vi "yaokong 10.23.vi"(0 "串口设置（遥控器）":T1={"波特率"=115200, "数据位"=8, "校验"=enum."None", "停止位"=10, "流控制"=0} {"流控制" items=["无"=0, "XON/XOFF"=1, "RTS/CTS"=2, "DTR/DSR"=4]; "停止位" items=["1.0"=10, "1.5"=15, "2.0"=20]; "数据位" min=5 max=8 step=1; "波特率" items=["460800"=460800, "75"=75, "110"=110, "134"=134, "150"=150, "300"=300, "600"=600, "1200"=1200, "1800"=1800, "2400"=2400, "4800"=4800, "7200"=7200, "9600"=9600, "14400"=14400, "19200"=19200, "28800"=28800, "38400"=38400, "56000"=56000, "57600"=57600, "115200"=115200, "128000"=128000, "230400"=230400]}, 2 "串口选择":refnum<visa-resource-name>="ASRL5::INSTR" caption="VISA资源名称") -> (9 "遥控器数据模式":T2={"CH0"=1024, "CH1"=1024, "CH2"=1024, "CH3"=1024, "CH5"=1024, "CH4"=1024, "Key0"=FALSE, "Key1"=FALSE, "Key2"=FALSE, "Key3"=FALSE, "Key4"=FALSE} {"CH4" scale=0.0..2048.0; "CH5" scale=0.0..2048.0; "CH3" scale=0.0..2048.0; "CH2" scale=0.0..2048.0; "CH1" scale=0.0..2048.0; "CH0" scale=0.0..2048.0})   [LabVIEW 2016]
uses:
  <vilib>/Platform/TimedLoop/XDataNode/timing_clust.ctl
  <vilib>/Platform/TimedLoop/XDataNode/nitl_modes.ctl
  <vilib>/Platform/TimedLoop/XDataNode/wakeup.ctl
  <vilib>/Instr/_visa.llb/VISA Configure Serial Port (Instr).vi
  <vilib>/imath/engines/lvmath2/RunTimeEngine/BuiltInFunctions/length/NIMS_length(GV).vi
  <instcachedir>/0/NIMS_length(GV)_08A3D13377FD4E4B96F5795FBF3698FA.lvgen/NIMS_length(GV)_08A3D13377FD4E4B96F5795FBF3698FA_003.vi
  <vilib>/imath/engines/lvmath2/RunTimeEngine/RangeToken/NIMS_Range_R3 - Integer.vi
  <instcachedir>/0/NIMS_Range_R3 - Integer_A435E2FF893B4C718FD5055FE39FE2F6.lvgen/NIMS_Range_R3 - Integer_A435E2FF893B4C718FD5055FE39FE2F6_000.vi
  <vilib>/imath/engines/lvmath2/RunTimeEngine/CommandStatement/MC_CommandStatement_break.vi
  <vilib>/imath/engines/lvmath2/RunTimeEngine/IndexRead/NIMS V(S).vi
  <instcachedir>/0/NIMS V(S)_0488751826AF41519A22953C041130DC.lvgen/NIMS V(S)_0488751826AF41519A22953C041130DC_004.vi
  <vilib>/imath/engines/lvmath2/RunTimeEngine/ErrorHandling/NIMS_Create Error From Enums.vi
  <vilib>/imath/engines/lvmath2/RunTimeEngine/RowToken/NIMS_RowToken_M_SorRV.vi
  <instcachedir>/0/NIMS_RowToken_M_SorRV_4D710C5E6F8040F3A39B2F03436798DB.lvgen/NIMS_RowToken_M_SorRV_4D710C5E6F8040F3A39B2F03436798DB_001.vi
  <vilib>/imathl/engines/lvmath/Functions/Error Handling/Create Error.vi
  <vilib>/imath/engines/lvmath2/RunTimeEngine/BuiltInFunctions/length/NIMS_length(GM).vi
  <instcachedir>/0/NIMS_length(GM)_47CEC356FCE0482D9BA47DC61C99F2C7.lvgen/NIMS_length(GM)_47CEC356FCE0482D9BA47DC61C99F2C7_001.vi
  <vilib>/imath/engines/lvmath2/RunTimeEngine/IndexRead/NIMS M(S).vi
  <instcachedir>/0/NIMS M(S)_B826C018497E4940AE96BD27B540B6FB.lvgen/NIMS M(S)_B826C018497E4940AE96BD27B540B6FB_005.vi
  <vilib>/imath/engines/lvmath2/RunTimeEngine/BuiltInFunctions/is_empty/NIMS_is_empty(GV).vi
  <instcachedir>/0/NIMS_is_empty(GV)_FC7E7C3D9544432CB6AA2416ADCF6D56.lvgen/NIMS_is_empty(GV)_FC7E7C3D9544432CB6AA2416ADCF6D56_000.vi
  <vilib>/imath/engines/lvmath2/RunTimeEngine/BuiltInFunctions/int32/NIMS_int32(int).vi
  <instcachedir>/0/NIMS_int32(int)_E7E4C8D9008A4CBD9466BF2F069BABE1.lvgen/NIMS_int32(int)_E7E4C8D9008A4CBD9466BF2F069BABE1_000.vi
  <vilib>/imath/engines/lvmath2/RunTimeEngine/BuiltInFunctions/is_empty/NIMS_is_empty(GM).vi
  <instcachedir>/0/NIMS_is_empty(GM)_AF8F13F4B7FD436CB1855477E2504B8A.lvgen/NIMS_is_empty(GM)_AF8F13F4B7FD436CB1855477E2504B8A_004.vi
  <vilib>/imath/engines/lvmath2/RunTimeEngine/BuiltInFunctions/zeros/NIMS_M=zeros(I32,I32).vi
  <vilib>/imath/engines/lvmath2/RunTimeEngine/IndexRead/NIMS V(R2).vi
  <instcachedir>/0/NIMS V(R2)_C76619605A0E4E9F8B2FA9389712AC47.lvgen/NIMS V(R2)_C76619605A0E4E9F8B2FA9389712AC47_002.vi
  <vilib>/imath/engines/lvmath2/RunTimeEngine/IndexReplace/NIMS M(S,$)=V.vi
  <instcachedir>/0/NIMS M(S,$)=V_BCCFA522A894489B8FA760383D74A164.lvgen/NIMS M(S,$)=V_BCCFA522A894489B8FA760383D74A164_001.vi
  <vilib>/imath/engines/lvmath2/RunTimeEngine/IndexRead/NIMS M($,S).vi
  <instcachedir>/0/NIMS M($,S)_3E5749BBB62E49528D4765A77F1F6D98.lvgen/NIMS M($,S)_3E5749BBB62E49528D4765A77F1F6D98_002.vi
  <vilib>/imath/engines/lvmath2/RunTimeEngine/BuiltInFunctions/sets_unique/NIMS_sets_unique(GV).vi
  <instcachedir>/0/NIMS_sets_unique(GV)_E0D8B80906AB4C8F84772F5CCB3705F2.lvgen/NIMS_sets_unique(GV)_E0D8B80906AB4C8F84772F5CCB3705F2_006.vi
  <instcachedir>/0/NIMS_length(GV)_08A3D13377FD4E4B96F5795FBF3698FA.lvgen/NIMS_length(GV)_08A3D13377FD4E4B96F5795FBF3698FA_002.vi
  <vilib>/imath/engines/lvmath2/RunTimeEngine/BuiltInFunctions/zeros/NIMS_V=zeros(I32,I32).vi
  <vilib>/imath/engines/lvmath2/RunTimeEngine/RangeToken/NIMS_Range_R2 - Integer.vi
  <instcachedir>/0/NIMS_Range_R2 - Integer_89B873E74E6E489885E44F751DD9C6BF.lvgen/NIMS_Range_R2 - Integer_89B873E74E6E489885E44F751DD9C6BF_000.vi
  <instcachedir>/0/NIMS V(S)_0488751826AF41519A22953C041130DC.lvgen/NIMS V(S)_0488751826AF41519A22953C041130DC_002.vi
  <vilib>/imath/engines/lvmath2/RunTimeEngine/BuiltInFunctions/sum/NIMS_sum(GV).vi
  <instcachedir>/0/NIMS_sum(GV)_67F5EC36BC034E54A6BEC5B0673C00E5.lvgen/NIMS_sum(GV)_67F5EC36BC034E54A6BEC5B0673C00E5_000.vi
  <vilib>/imath/engines/lvmath2/RunTimeEngine/IndexReplace/NIMS V(S)=S.vi
  <instcachedir>/0/NIMS V(S)=S_57E16554CB8B4B90AAB163894F717546.lvgen/NIMS V(S)=S_57E16554CB8B4B90AAB163894F717546_000.vi
  <vilib>/imath/engines/lvmath2/RunTimeEngine/BuiltInFunctions/max/1 input/NIMS_max(RV).vi
  <instcachedir>/0/NIMS_max(RV)_237633DB1D604D5BA7001287DF3C7957.lvgen/NIMS_max(RV)_237633DB1D604D5BA7001287DF3C7957_000.vi
  <vilib>/imath/engines/lvmath2/RunTimeEngine/BuiltInFunctions/findnz/NIMS_[1o]_findnz(GRowV).vi
  <instcachedir>/0/NIMS_[1o]_findnz(GRowV)_1AF74843B4874134ADE908C0A4A72F3C.lvgen/NIMS_[1o]_findnz(GRowV)_1AF74843B4874134ADE908C0A4A72F3C_000.vi
  <vilib>/imath/engines/lvmath2/RunTimeEngine/IndexRead/NIMS M($,R2).vi
  <instcachedir>/0/NIMS M($,R2)_D9380E19261A4ADFB2D364AF6959C6EF.lvgen/NIMS M($,R2)_D9380E19261A4ADFB2D364AF6959C6EF_002.vi
  <vilib>/imath/engines/lvmath2/RunTimeEngine/BuiltInFunctions/median/NIMS_RRow=median(RM,I32).vi
  <vilib>/imath/engines/lvmath2/RunTimeEngine/BuiltInFunctions/int32/NIMS_int32(real).vi
  <instcachedir>/0/NIMS_int32(real)_9F6AE75EF4BE45429513317A1C5A7040.lvgen/NIMS_int32(real)_9F6AE75EF4BE45429513317A1C5A7040_002.vi
  <vilib>/imath/engines/lvmath2/RunTimeEngine/VariableToken/NIMS_VariableToken_CondDefined.vi
  <instcachedir>/0/NIMS_VariableToken_CondDefined_06E9DA95BD4D46A6BA55EC651A891960.lvgen/NIMS_VariableToken_CondDefined_06E9DA95BD4D46A6BA55EC651A891960_004.vi
  <vilib>/imath/engines/lvmath2/RunTimeEngine/NodeEndStatement/NIMS_NodeEndStatement_Get Vector.vi
  <instcachedir>/0/NIMS_NodeEndStatement_Get Vector_9E4547DF38A84F62A7E036B4CE3D251C.lvgen/NIMS_NodeEndStatement_Get Vector_9E4547DF38A84F62A7E036B4CE3D251C_002.vi
  <vilib>/imath/engines/lvmath/Functions/Error Handling/MergeErrorsWrapper.vi
  <vilib>/imath/engines/lvmath2/RunTimeEngine/NodeEndStatement/NIMS_NodeEndStatement_Output.vi
  <instcachedir>/0/NIMS_NodeEndStatement_Output_53EC0D466D134D7ABD903AC30B43404B.lvgen/NIMS_NodeEndStatement_Output_53EC0D466D134D7ABD903AC30B43404B_004.vi
  <instcachedir>/0/NIMS_NodeEndStatement_Output_53EC0D466D134D7ABD903AC30B43404B.lvgen/NIMS_NodeEndStatement_Output_53EC0D466D134D7ABD903AC30B43404B_010.vi
  <vilib>/imath/engines/lvmath2/RunTimeEngine/ErrorHandling/NIMS_Finalize Error.vi
  <vilib>/Platform/TimedLoop/XDataNode/XDataNode.xnode
  <vilib>/Platform/TimedLoop/XDataNode/XDNodeRunTimeDep.lvlib
panel:
  out "error out":errorcluster caption="错误输出"
  in  "遥控器数据队列名":string="Queue_RemoteCtler"
  out "CtlerFrameData":u8[](array[numeric])
  out "输出变量":i32
  in  "全局停止":bool
  out "Serial Settings:Number of Bytes at Serial Port":u32
  out "CtlerData":u8[](array[numeric])
  out "读取缓冲区":string
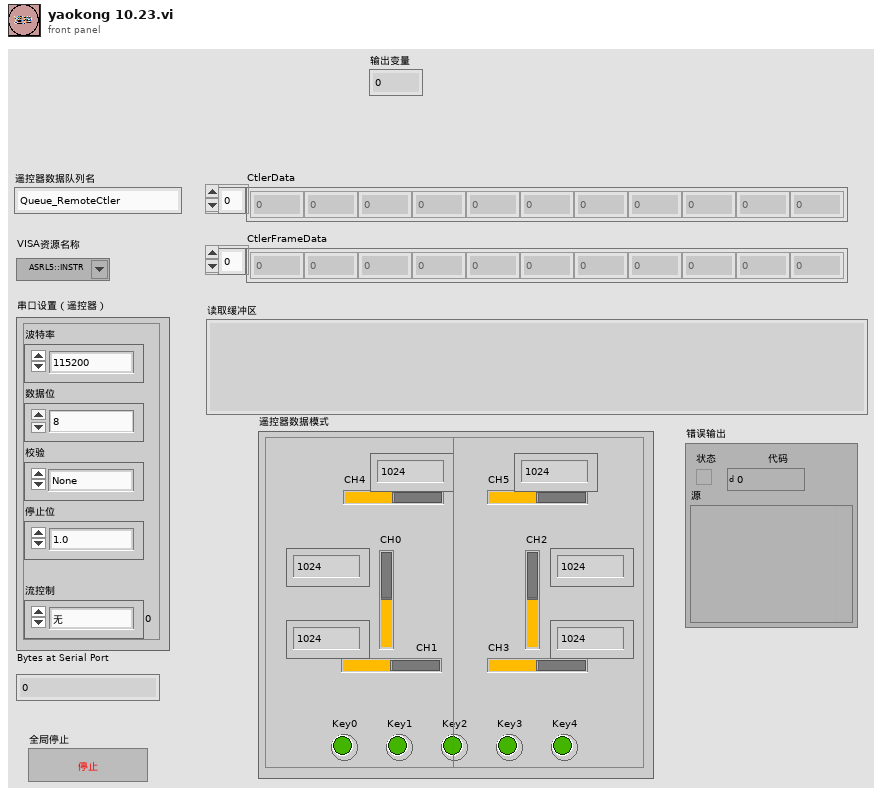
[diagram p1: front panel]
types:
  T1 = cluster{"波特率":u32, "数据位":u16, "校验":enum16{"None", "Odd", "Even", "Mark", "Space"}, "停止位":u16, "流控制":u16}
  T2 = cluster{"CH0":i32, "CH1":i32, "CH2":i32, "CH3":i32, "CH5":i32, "CH4":i32, "Key0":bool, "Key1":bool, "Key2":bool, "Key3":bool, "Key4":bool}
  T3 = typedef "XDNodeRunTimeDep.lvlib/timing_clust.ctl" = cluster{"Expected End [f-1]":u64, "Actual End [f-1]":u64, "Finished Late? [f-1]":bool, "Expected End [i-1]":u64, "Actual End [i-1]":u64, "Finished Late? [i-1]":bool, "Expected Start [i]":u64, "Actual Start [i]":u64, "Expected Start [f]":u64, "Actual Start [f]":u64, "Source Name":string, "Structure Name":string, "Period":i64, "Deadline":i64, "Offset":i64, "Start":i64, "Priority":i32, "Timeout":i32, "Mode":T4, "Wakeup Reason":T5, "Error":errorcluster, "Source Type":string, "Secondary Source Type":string, "Global End Time":u64, "Global Start Time":u64, "Frame Duration":u64, "Iteration Duration":u64, "Assigned CPU":i32, "I/O Scan Engine Mode":u32}
  T4 = typedef "XDNodeRunTimeDep.lvlib/nitl_modes.ctl" = enum32{"No Change", "Process missed periods, maintain original phase", "Discard missed periods, maintain original phase", "Process missed periods, ignore original phase", "Discard missed periods, ignore original phase"}
  T5 = typedef "XDNodeRunTimeDep.lvlib/wakeup.ctl" = enum32{"Normal", "Aborted", "Asynchronous wakeup", "Timing source error", "Timed loop error", "Timeout"}
  T6 = cluster{i32, i32, i32, i32, i32, i32, bool, bool, bool, bool, bool}
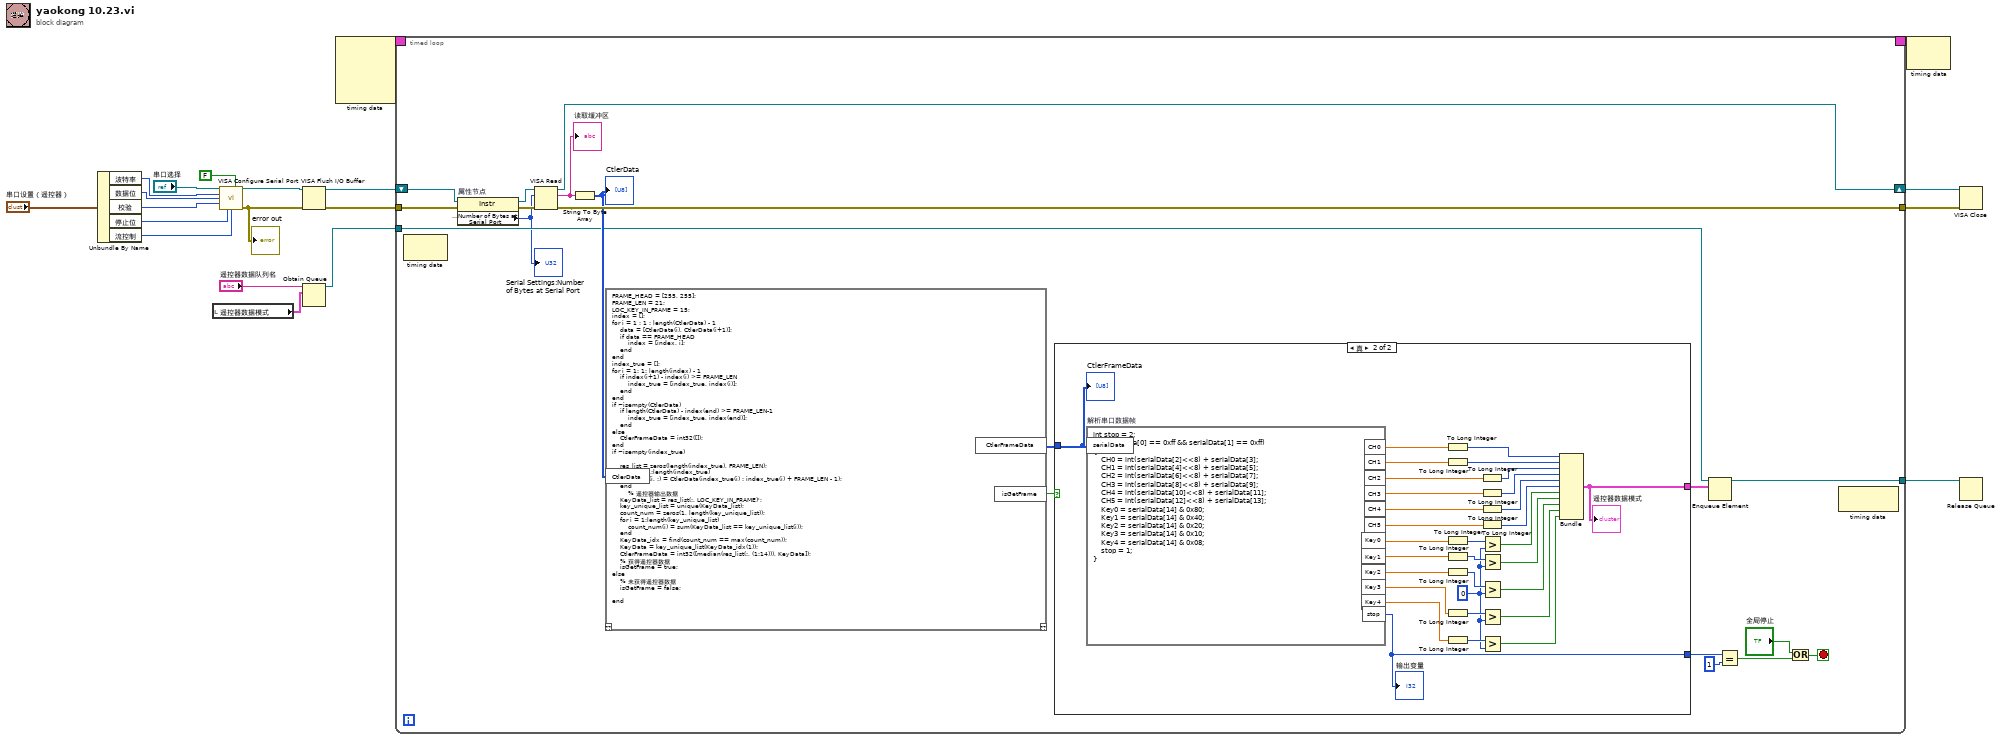
[diagram p0: block diagram]
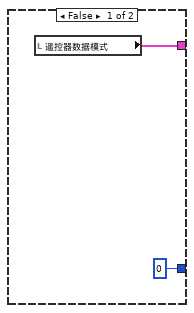
[diagram p2: hidden frame]
diagram:
  n1 = Unbundle By Name("串口设置（遥控器）") -> ("波特率"=w17:u32, "数据位"=w16:u16, "校验"=w15:enum16{"None", "Odd", "Even", "Mark", "Space"}, "停止位"=w14:u16, "流控制"=w13:u16)
  n2 = local read "遥控器数据模式"() -> (w6:T2)
  n3 = call-poly "VISA Configure Serial Port"("VISA resource name"="串口选择", "Enable Termination\nChar (T)"=FALSE ("Enable Termination\nChar (T)"), "baud rate (9600)"=w17, "data bits (8)"=w16, "parity (0:none)"=w15, "stop bits (10: 1 bit)"=w14, "flow control (0:none)"=w13) -> ("VISA resource name out"=w4:refnum<visa-resource-name>, "error out"=w3:errorcluster)  [unwired: 2 in, 5 out]
  "error out" <- w3
  n4 = VISA Flush I/O Buffer(VISA resource name=w4, error in (no error)=w3) -> (VISA resource name out=w1:refnum<visa-resource-name>, error out=w2:errorcluster)  [unwired: 1 in]
  n5 = Obtain Queue(name (unnamed)="遥控器数据队列名", element data type=w6) -> (queue out=w8:refnum<queue>)  [unwired: 3 in, 2 out]
  n6 = node-c288() -> (w20:T3)  [unwired: 4 in]
  n7 = timed-loop {
    tunnel: w2 -> [w38]
    shift-right: [w35] -> w11
    shift-left: w1 -> [w39]
    tunnel: [w34] -> w10
    tunnel: w8 -> [w30]
    tunnel: [w29] -> w7
    timing: w20 -> [_]
    timing-out: [_] -> w19
    stop <- w21 stop-if-true
    n8 = node-c288() -> ()  [unwired: 1 in, 1 out]
    n9 = property on="属性节点" class="Instr"(reference=w39, error in=w38) -> (reference out=w37:refnum<visa-resource-name>, error out=w36:errorcluster, "Serial Settings:Number of Bytes at Serial Port"=w28:u32)
    "Serial Settings:Number of Bytes at Serial Port" <- w28
    n10 = VISA Read(VISA resource name=w37, byte count=w28, error in (no error)=w36) -> (VISA resource name out=w35:refnum<visa-resource-name>, read buffer=w33:string, error out=w34:errorcluster)  [unwired: 1 out]
    "读取缓冲区" <- w33
    n11 = String To Byte Array(string=w33) -> (unsigned byte array=w32:u8[])
    "CtlerData" <- w32
    n12 = mathscript code="FRAME_HEAD = [255, 255];\nFRAME_LEN = 21;\nLOC_KEY_IN_FRAME = 15;\nindex = [];\nfor i = 1 : 1 : length(CtlerData) - 1\n    data = [CtlerData(i), CtlerData(i+1)];\n    if data == FRAME_HEAD\n        index = [index, i]; \n    end\nend\nindex_true = [];\nfor i = 1: 1: length(index) - 1\n    if index(i+1) - index(i) >= FRAME_LEN\n        index_true = [index_true, index(i)];\n    end\nend\nif ~isempty(CtlerData)\n    if length(CtlerData) - index(end) >= FRAME_LEN-1\n        index_true = [index_true, index(end)];\n    end\nelse\n    CtlerFrameData = int32([]);\nend\nif ~isempty(index_true)\n    \n    res_list = zeros(length(index_true), FRAME_LEN);\n    for i = 1:1:length(index_true)\n        res_list(i, :) = CtlerData(index_true(i) : index_true(i) + FRAME_LEN - 1);\n    end\n        % 遥控器输出数据\n    KeyData_list = res_list(:, LOC_KEY_IN_FRAME)';\n    key_unique_list = unique(KeyData_list);\n    count_num = zeros(1, length(key_unique_list));\n    for i = 1:length(key_unique_list)\n        count_num(i) = sum(KeyData_list == key_unique_list(i));\n    end\n    KeyData_idx = find(count_num == max(count_num));\n    KeyData = key_unique_list(KeyData_idx(1));\n    CtlerFrameData = int32([median(res_list(:, (1:14))), KeyData]);\n    % 获得遥控器数据\n    isGetFrame = true;\nelse\n    % 未获得遥控器数据\n    isGetFrame = false;\n   \nend"("CtlerData"=w32) -> ("CtlerFrameData"=w27:i32[], "isGetFrame"=w31:bool)  [unwired: 1 in, 1 out]
    n13 = case shown="真" w31 {
      tunnel: [w740 w744] -> w26
      tunnel: w27 -> [_ w742]
      tunnel: [0 ("y") w741] -> w25
      frame False {
        n14 = local read "遥控器数据模式"() -> (w740:T2)
      }
      frame True {
        w745 = 0 ("y")
        n15 = formula code="int stop = 2;\nif (serialData[0] == 0xff && serialData[1] == 0xff)\n{\n    CH0 = int(serialData[2]<<8) + serialData[3];\n    CH1 = int(serialData[4]<<8) + serialData[5];\n    CH2 = int(serialData[6]<<8) + serialData[7];\n    CH3 = int(serialData[8]<<8) + serialData[9];\n    CH4 = int(serialData[10]<<8) + serialData[11];\n    CH5 = int(serialData[12]<<8) + serialData[13];\n    Key0 = serialData[14] & 0x80;\n    Key1 = serialData[14] & 0x40;\n    Key2 = serialData[14] & 0x20;\n    Key3 = serialData[14] & 0x10;\n    Key4 = serialData[14] & 0x08;\n    stop = 1;\n}" "解析串口数据帧"("serialData"=w742) -> ("CH0"=w771:dbl, "CH1"=w770:dbl, "CH2"=w769:dbl, "CH3"=w768:dbl, "CH4"=w767:dbl, "CH5"=w766:dbl, "Key0"=w765:dbl, "Key1"=w764:dbl, "Key2"=w763:dbl, "Key3"=w762:dbl, "Key4"=w761:dbl, "stop"=w741:i32)
        "输出变量" <- w741
        n16 = To Long Integer(number=w771) -> (32bit integer=w743:i32)
        n17 = To Long Integer(number=w770) -> (32bit integer=w760:i32)
        n18 = To Long Integer(number=w765) -> (32bit integer=w755:i32)
        n19 = To Long Integer(number=w764) -> (32bit integer=w746:i32)
        n20 = To Long Integer(number=w763) -> (32bit integer=w752:i32)
        n21 = To Long Integer(number=w762) -> (32bit integer=w749:i32)
        n22 = To Long Integer(number=w761) -> (32bit integer=w747:i32)
        n23 = To Long Integer(number=w769) -> (32bit integer=w759:i32)
        n24 = To Long Integer(number=w768) -> (32bit integer=w758:i32)
        n25 = To Long Integer(number=w767) -> (32bit integer=w757:i32)
        n26 = To Long Integer(number=w766) -> (32bit integer=w756:i32)
        n27 = Greater?(x=w755, y=w745) -> (0:w754:bool)
        n28 = Greater?(x=w746, y=w745) -> (0:w753:bool)
        n29 = Greater?(x=w752, y=w745) -> (0:w751:bool)
        n30 = Greater?(x=w749, y=w745) -> (0:w750:bool)
        n31 = Greater?(x=w747, y=w745) -> (0:w748:bool)
        n32 = Bundle(w743, w760, w759, w758, w757, w756, w754, w753, w751, w750, w748) -> (w744:T6)  [unwired: 1 in]
        "遥控器数据模式" <- w744
        "CtlerFrameData" <- w742
      }
    }
    n33 = Enqueue Element(queue=w30, element=w26) -> (queue out=w29:refnum<queue>)  [unwired: 2 in, 2 out]
    n34 = Equal?(x=w25, y=1) -> (x = y?=w23:bool)
    n35 = Or(x="全局停止", y=w23) -> (x .or. y?=w21:bool)
    n36 = node-c288() -> ()  [unwired: 1 in, 1 out]
  }
  n37 = node-c288(w19) -> ()  [unwired: 1 out]
  n38 = VISA Close(VISA resource name=w11, error in (no error)=w10) -> ()  [unwired: 1 out]
  n39 = Release Queue(queue=w7) -> ()  [unwired: 2 in, 3 out]
